vi "System Log.vi"(8 "error in (no error)":errorcluster, 10 "Text to log":string, 11 "uService Template in":refnum<class "Father of all uServices.lvclass">) -> (0 "error out":errorcluster, 3 "uService Template out":refnum<class "Father of all uServices.lvclass">)   [LabVIEW 2026, in "TALOS.lvlib" / "Father of all uServices.lvlib" / "Father of all uServices.lvclass"]
doc: "Log the text in the system log."
uses:
  Father of all uServices.lvclass
  TALOS.lvlib
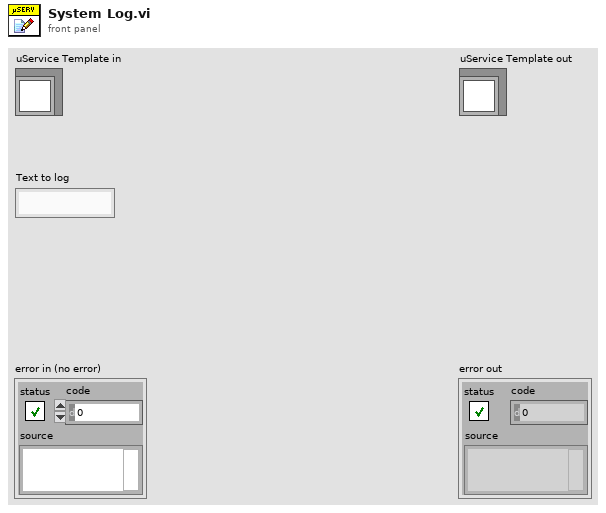
[diagram p1: front panel]
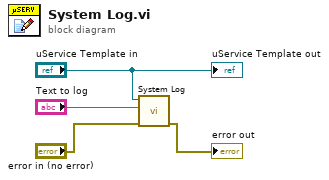
[diagram p0: block diagram]
diagram:
  n1 = call "System Log.vi"("error in (no error)"="error in (no error)", "Text to log"="Text to log", "Object in"="uService Template in") -> ("error out"=→"error out":errorcluster)  [unwired: 8 in]
  "uService Template out" <- "uService Template in"
